vi "CheckSettingsFolder.vi"() -> ()   [LabVIEW 2022 SP3]
panel:
  out "text":string
  out "DataPath Out":path
  out "files":string[](array[string])
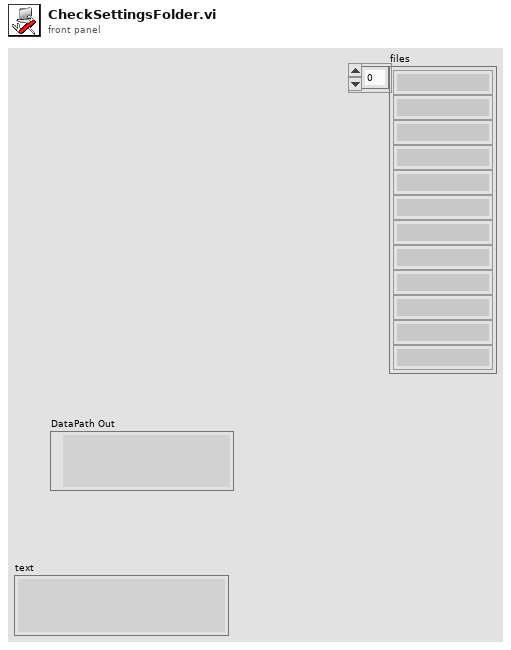
[diagram p1: front panel]
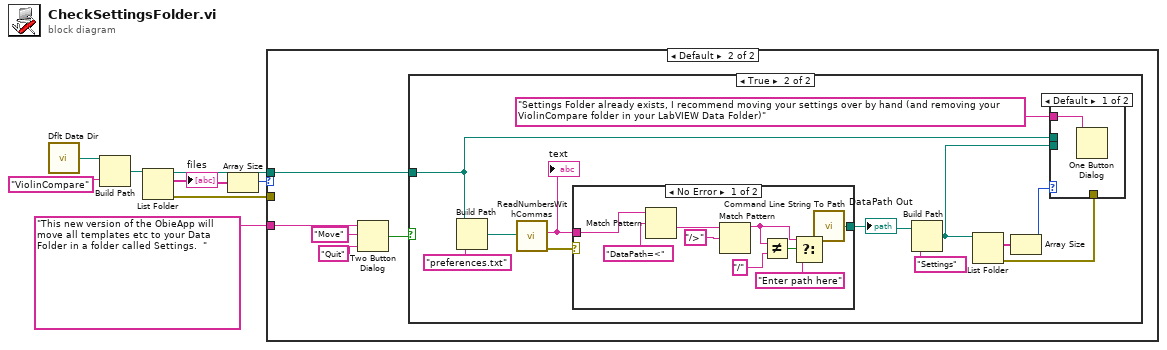
[diagram p0: block diagram]
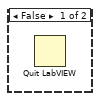
[diagram p3: hidden frame]
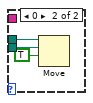
[diagram p4: hidden frame]
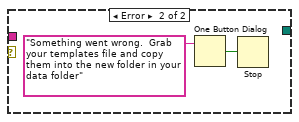
[diagram p5: hidden frame]
diagram:
  n1 = call <vilib>:"Dflt Data Dir.vi"() -> ("App:Default Data Directory"=w7:path)
  n2 = Build Path(base path=w7, name or relative path="ViolinCompare") -> (appended path=w6:path)
  n3 = List Folder(path=w6) -> (path out=w3:path, filenames=w5:string[], error out=w2:errorcluster)  [unwired: 3 in, 1 out]
  "files" <- w5
  n4 = Array Size(array=w5) -> (size(s)=w4:i32)
  n5 = case shown="Default" w4 {
    tunnel: w3 -> [_ w13]
    tunnel: w2 -> [_ _]
    tunnel: "This new version of the ObieApp will move all templates etc to your Data Folder in a folder called Settings.  " ("name or relative path") -> [_ w12]
    frame 0 {
    }
    frame Default {
      n6 = Two Button Dialog(message=w12, 1:"Quit" ("F button name (\"Cancel\")"), 2:"Move" ("T button name (\"OK\")")) -> (T button?=w11:bool)
      n7 = case shown="True" w11 {
        tunnel: w13 -> [_ w24]
        frame False {
          n8 = Quit LabVIEW() -> ()  [unwired: 1 in]
        }
        frame True {
          n9 = Build Path(base path=w24, name or relative path="preferences.txt") -> (appended path=w16:path)
          n10 = call "ReadNumbersWithCommas.vi"("file (use dialog)"=w16) -> ("error out"=w14:errorcluster, "text"=w15:string)  [unwired: 7 in, 2 out]
          "text" <- w15
          n11 = case shown="No Error" w14 {
            tunnel: [w39 _] -> w22
            tunnel: w15 -> [w38 _]
            frame No Error {
              n12 = Match Pattern(string=w38, regular expression="DataPath=<" ("format string")) -> (after substring=w37:string)  [unwired: 1 in, 3 out]
              n13 = Match Pattern(string=w37, regular expression="/>" ("format string")) -> (before substring=w32:string)  [unwired: 1 in, 3 out]
              n14 = Not Equal?(x=w32, y="/" ("format string")) -> (x != y?=w33:bool)
              n15 = Select(t=w32, s=w33, f="Enter path here" ("format string")) -> (s? t:f=w31:string)
              n16 = call <vilib>:"Command Line String To Path.vi"("string"=w31) -> ("path"=w39:path)
            }
            frame Error {
              n17 = One Button Dialog(message="Something went wrong.  Grab your templates file and copy them into the new folder in your data folder") -> (true=w41:bool)  [unwired: 1 in]
              n18 = Stop(stop? (T)=w41) -> ()
            }
          }
          "DataPath Out" <- w22
          n19 = Build Path(base path=w22, name or relative path="Settings") -> (appended path=w21:path)
          n20 = List Folder(path=w21) -> (filenames=w20:string[], error out=w18:errorcluster)  [unwired: 3 in, 2 out]
          n21 = Array Size(array=w20) -> (size(s)=w19:i32)
          n22 = case shown="Default" w19 {
            tunnel: w24 -> [_ w29]
            tunnel: w21 -> [_ w27]
            tunnel: w18 -> [_ _]
            tunnel: "Settings Folder already exists, I recommend moving your settings over by hand (and removing your ViolinCompare folder in your LabVIEW Data Folder)" ("name or relative path") -> [w26 _]
            frame Default {
              n23 = One Button Dialog(message=w26) -> ()  [unwired: 1 in, 1 out]
            }
            frame 0 {
              n24 = Move(source path=w29, 9:TRUE ("overwrite (F)"), 10:w27) -> ()  [unwired: 2 in, 3 out]
            }
          }
        }
      }
    }
  }
